vi "Hardware - Access Analog Data Queue.vi"(7 "Method":T2=enum."Preview Element", 8 "error in (no error)":errorcluster, 9 "timeout in ms (-1)":i32=-1, 11 "Analog Data Queue":refnum<queue>) -> (0 "error out":errorcluster, 1 "Analog Data Out":refnum<queue>, 2 "timed out?":bool, 3 "Analog Data":T1)   [LabVIEW 2010, in "Core SubVIs.lvlib"]
uses:
  Core SubVIs.lvlib
  Controls/TYPE - Analog Data.ctl
  Controls/TYPE - Analog Data Queue Method.ctl
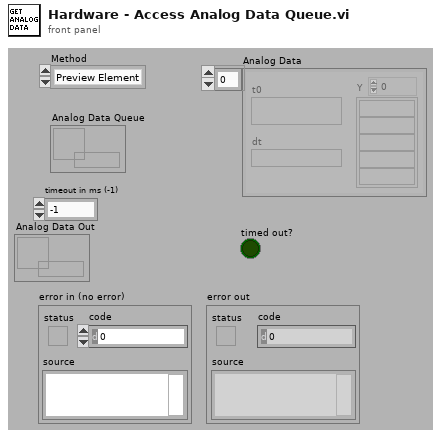
[diagram p1: front panel]
types:
  T1 = typedef "Core SubVIs.lvlib/TYPE - Analog Data.ctl" = waveform(dbl)[]
  T2 = typedef "Core SubVIs.lvlib/TYPE - Analog Data Queue Method.ctl" = enum16{"Set Data Queue", "Preview Element", "Remove Element", "Get Data Queue", "Flush Data Queue"}
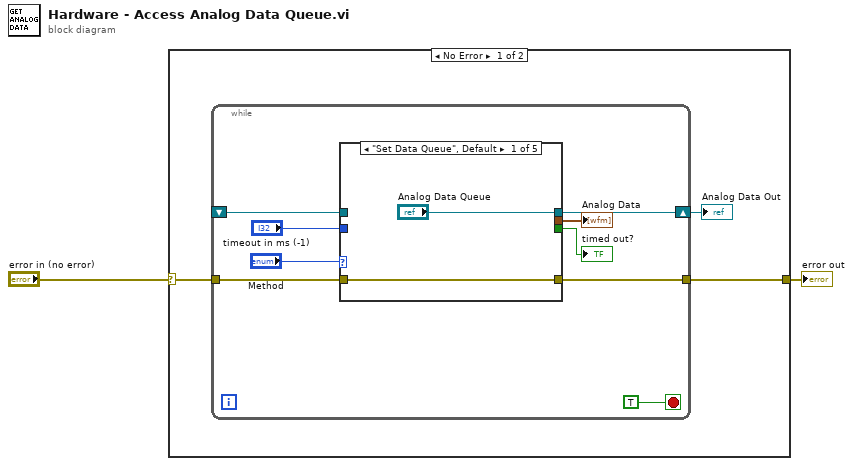
[diagram p0: block diagram]
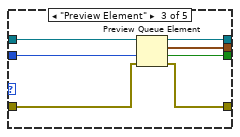
[diagram p3: hidden frame]
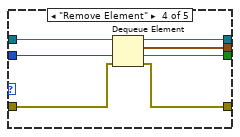
[diagram p4: hidden frame]
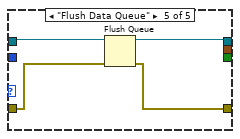
[diagram p5: hidden frame]
diagram:
  n1 = case shown="No Error" "error in (no error)" {
    selector: "error in (no error)" -> [w5 w37]
    tunnel: [w4 w37] -> w1
    frame No Error {
      n2 = while {
        shift-right: [w14] -> w3
        shift-left: _ -> [w12]
        tunnel: w5 -> [w8]
        tunnel: [w7] -> w4
        stop <- TRUE stop-if-true
        n3 = case shown="\"Set Data Queue\", Default" "Method" {
          tunnel: w12 -> [_ w17 w25 w32 w36]
          tunnel: ["Analog Data Queue" w17 w24 w31 w35] -> w14
          tunnel: [_ _ w23 w30 _] -> w11
          tunnel: [_ _ w22 w29 _] -> w10
          tunnel: w8 -> [w15 w18 w21 w28 w33]
          tunnel: [w15 w18 w20 w27 w34] -> w7
          tunnel: "timeout in ms (-1)" -> [_ _ w19 w26 _]
          frame "Set Data Queue", Default {
          }
          frame "Get Data Queue" {
          }
          frame "Preview Element" {
            n4 = Preview Queue Element(queue=w25, timeout in ms (-1)=w19, error in (no error)=w21) -> (queue out=w24:refnum<queue>, element=w23:T1, timed out?=w22:bool, error out=w20:errorcluster)
          }
          frame "Remove Element" {
            n5 = Dequeue Element(queue=w32, timeout in ms (-1)=w26, error in (no error)=w28) -> (queue out=w31:refnum<queue>, element=w30:T1, timed out?=w29:bool, error out=w27:errorcluster)
          }
          frame "Flush Data Queue" {
            n6 = Flush Queue(queue=w36, error in (no error)=w33) -> (queue out=w35:refnum<queue>, error out=w34:errorcluster)  [unwired: 1 out]
          }
        }
        "Analog Data" <- w11
        "timed out?" <- w10
      }
      "Analog Data Out" <- w3
    }
    frame Error {
    }
  }
  "error out" <- w1
